vi "V2-adam-write-&-check-response.vi"(8 "error in (no error)":errorcluster, 10 "write buffer":string, 11 "VISA resource name":refnum<visa-resource-name>) -> (0 "error out":errorcluster, 1 "cmd aknowledged":bool, 2 "acknowledge char":string, 3 "VISA resource name out":refnum<visa-resource-name>, 4 "read buffer":string)   [LabVIEW 2024]
panel:
  out "return count":u32
  out "number pause loops":i32
  out "No. Bytes at Port":u32
  out "read return":u32
  out "pause-time":u32
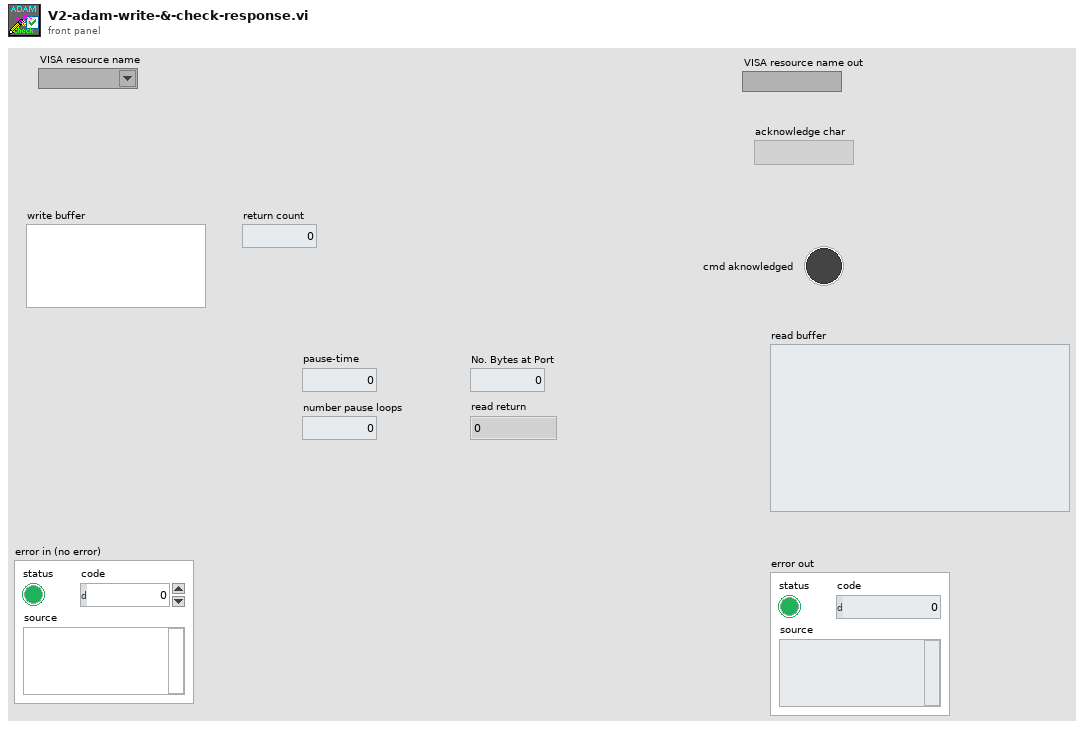
[diagram p1: front panel]
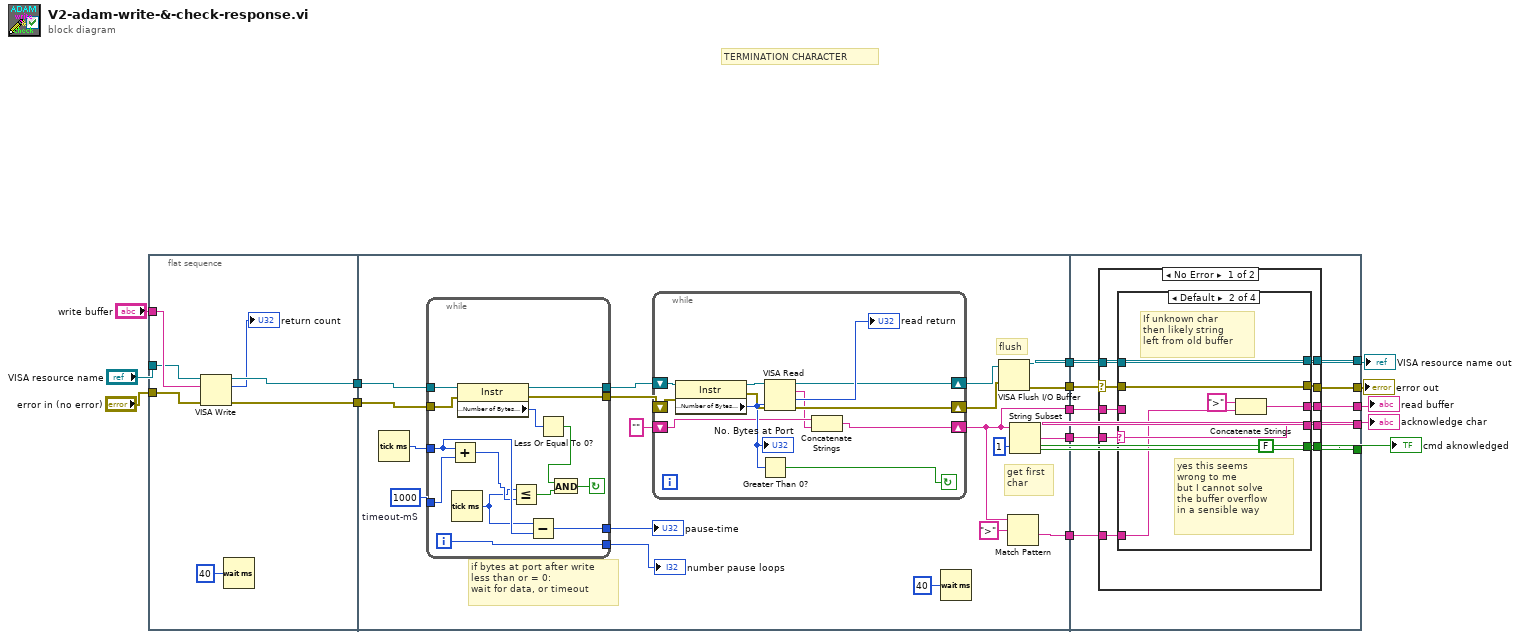
[diagram p0: block diagram]
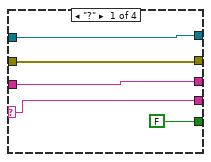
[diagram p2: hidden frame]
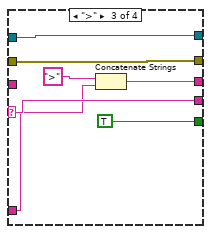
[diagram p3: hidden frame]
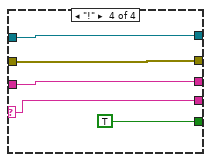
[diagram p4: hidden frame]
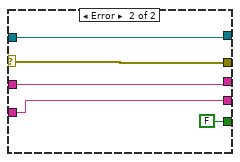
[diagram p5: hidden frame]
diagram:
  # "TERMINATION CHARACTER"
  n1 = flat-sequence {
    tunnel: "error in (no error)" -> [w20]
    tunnel: "VISA resource name" -> [w21]
    tunnel: "write buffer" -> [w22]
    tunnel: [w19] -> w5
    tunnel: [w18] -> w4
    tunnel: [w26] -> w12
    tunnel: [w40] -> w11
    tunnel: [w39] -> w10
    tunnel: w5 -> [w35]
    tunnel: w4 -> [w34]
    tunnel: [w25] -> w3
    tunnel: [w24] -> w1
    tunnel: w12 -> [w76]
    tunnel: w11 -> [w77]
    tunnel: w10 -> [w75]
    tunnel: [w74] -> w9
    tunnel: [w73] -> w8
    tunnel: [w72] -> w7
    tunnel: [w71] -> w6
    tunnel: w3 -> [w70]
    tunnel: [w69] -> w2
    tunnel: w1 -> [w68]
    frame #0 {
      n2 = VISA Write(VISA resource name=w21, write buffer=w22, error in (no error)=w20) -> (VISA resource name out=w18:refnum<visa-resource-name>, return count=→"return count":u32, error out=w19:errorcluster)
      n3 = Wait (ms)(milliseconds to wait=u32 40) -> ()  [unwired: 1 out]
    }
    frame #1 {
      w37 = u32 1000  # timeout-mS
      # "if bytes at port after write\nless than or = 0:\nwait for data, or timeout"
      # "get first\nchar"
      # "flush"
      n4 = Tick Count (ms)() -> (millisecond timer value=w38:u32)
      n5 = while {
        tunnel: [w67] -> w32
        tunnel: [w66] -> w31
        tunnel: w38 -> [w61]
        tunnel: w37 -> [w65]
        tunnel: [w60] -> w36
        tunnel: w35 -> [w59]
        tunnel: w34 -> [w58]
        tunnel: [w57] -> w33
        i -> [w57]
        stop <- w64 continue-if-true
        n6 = Add(x=w61, y=w65) -> (x+y=w56:u32)
        n7 = Tick Count (ms)() -> (millisecond timer value=w55:u32)
        n8 = property class="Instr"(reference=w58, error in=w59) -> (reference out=w67:refnum<visa-resource-name>, error out=w66:errorcluster, "Serial Settings:Number of Bytes at Serial Port"=w54:u32)
        n9 = Less Or Equal?(x=w55, y=w56) -> (x <= y?=w62:bool)
        n10 = Subtract(x=w55, y=w61) -> (x-y=w60:u32)
        n11 = Less Or Equal To 0?(x=w54) -> (x <= 0?=w63:bool)
        n12 = And(x=w63, y=w62) -> (x .and. y?=w64:bool)
      }
      "pause-time" <- w36
      "number pause loops" <- w33
      n13 = while {
        shift-right: [w47] -> w30
        shift-left: w32 -> [w49]
        shift-right: [w46] -> w29
        shift-left: w31 -> [w48]
        shift-right: [w43] -> w24
        shift-left: "" ("read buffer") -> [w45]
        stop <- w42 continue-if-true
        n14 = property class="Instr"(reference=w49, error in=w48) -> (reference out=w52:refnum<visa-resource-name>, error out=w53:errorcluster, "Serial Settings:Number of Bytes at Serial Port"=w50:u32)
        "No. Bytes at Port" <- w50
        n15 = Greater Than 0?(x=w50) -> (x > 0?=w42:bool)
        n16 = VISA Read(VISA resource name=w52, byte count=w50, error in (no error)=w53) -> (VISA resource name out=w47:refnum<visa-resource-name>, read buffer=w44:string, return count=→"read return":u32, error out=w46:errorcluster)
        n17 = Concatenate Strings(w45, w44) -> (w43:string)
      }
      n18 = Wait (ms)(milliseconds to wait=u32 40) -> ()  [unwired: 1 out]
      n19 = VISA Flush I/O Buffer(VISA resource name=w30, error in (no error)=w29) -> (VISA resource name out=w39:refnum<visa-resource-name>, error out=w40:errorcluster)  [unwired: 1 in]
      n20 = Match Pattern(string=w24, regular expression=">") -> (after substring=w25:string)  [unwired: 1 in, 3 out]
      n21 = String Subset(string=w24, length (rest)=1 ("length (rest)")) -> (substring=w26:string)  [unwired: 1 in]
    }
    frame #2 {
      n22 = case shown="No Error" w77 {
        selector: w77 -> [w83 w116]
        tunnel: [w87 FALSE ("cmd aknowledged")] -> w74
        tunnel: w76 -> [w86 w115]
        tunnel: [w85 w115] -> w73
        tunnel: [w84 w116] -> w72
        tunnel: w75 -> [w82 w113]
        tunnel: [w81 w113] -> w71
        tunnel: w70 -> [w80 _]
        tunnel: [w79 w112] -> w69
        tunnel: w68 -> [w78 w112]
        frame No Error {
          n23 = case shown="Default" w86 {
            selector: w86 -> [w91 w98 w105 w110]
            tunnel: [FALSE ("cmd aknowledged") FALSE ("cmd aknowledged") TRUE ("cmd aknowledged") TRUE ("cmd aknowledged")] -> w87
            tunnel: [w91 w98 w105 w110] -> w85
            tunnel: [w90 w97 w104 w109] -> w84
            tunnel: w83 -> [w90 w97 w104 w109]
            tunnel: w82 -> [w89 w96 w103 w108]
            tunnel: [w89 w96 w103 w108] -> w81
            tunnel: w80 -> [_ w94 w102 _]
            tunnel: [w88 w95 w101 w107] -> w79
            tunnel: w78 -> [w88 _ _ w107]
            frame "?" {
            }
            frame Default {
              # "yes this seems\nwrong to me\nbut I cannot solve \nthe buffer overflow \nin a sensible way"
              # "If unknown char\nthen likely string\nleft from old buffer"
              n24 = Concatenate Strings(">" ("string"), w94) -> (w95:string)
            }
            frame ">" {
              n25 = Concatenate Strings(">" ("string"), w102) -> (w101:string)
            }
            frame "!" {
            }
          }
        }
        frame Error {
        }
      }
    }
  }
  "error out" <- w7
  "VISA resource name out" <- w6
  "cmd aknowledged" <- w9
  "acknowledge char" <- w8
  "read buffer" <- w2
